vi "test_PhotonPoseEstimator_lowestAmbiguity.vi"(8 "error in (no error)":errorcluster) -> (0 "error out":errorcluster, 3 "Test Passed":bool)   [LabVIEW 2019]
uses:
  <vilib>/Rock Robotics/WPI/ThirdParty/PhotonVisionLib/TypeDef/PhotonEstimatedRobotPoseType.ctl
  <vilib>/Rock Robotics/WPI/ThirdParty/JAS_Junk/TrajLib/TypeDef/POSE3D.ctl
  <vilib>/Rock Robotics/WPI/ThirdParty/JAS_Junk/TrajLib/TypeDef/TRANSLATION3D.ctl
  <vilib>/Rock Robotics/WPI/ThirdParty/JAS_Junk/TrajLib/TypeDef/ROTATION3D.ctl
  <vilib>/Rock Robotics/WPI/ThirdParty/JAS_Junk/TrajLib/TypeDef/QUATERNION.ctl
  <vilib>/Rock Robotics/WPI/ThirdParty/PhotonVisionLib/TypeDef/PhotonPoseStrategy_ENUM.ctl
  <vilib>/Rock Robotics/WPI/ThirdParty/JAS_Junk/TrajLib/VI/Translation3d_Create_Default.vi
  <vilib>/Rock Robotics/WPI/ThirdParty/JAS_Junk/TrajLib/VI/Rotation3d_Create_Default.vi
  <vilib>/Rock Robotics/WPI/ThirdParty/JAS_Junk/TrajLib/VI/Quaternion_New.vi
  <vilib>/Rock Robotics/WPI/ThirdParty/PhotonVisionLib/SubVI/PhotonPipelineResult_HasTargets.vi
  <vilib>/Rock Robotics/WPI/ThirdParty/PhotonVisionLib/SubVI/PhotonEstimatedRobotPose_New.vi
  <vilib>/Rock Robotics/WPI/ThirdParty/PhotonVisionLib/SubVI/PhotonPipelineResult_GetTargets.vi
  <vilib>/Rock Robotics/WPI/ThirdParty/PhotonVisionLib/SubVI/PhotonTrackedTarget_GetPoseAmbiguity.vi
  <vilib>/Rock Robotics/WPI/ThirdParty/PhotonVisionLib/SubVI/PhotonTrackedTarget_GetFiducialId.vi
  <vilib>/Rock Robotics/WPI/ThirdParty/PhotonVisionLib/SubVI/PhotonPoseEstimator_GetFieldTags.vi
  <vilib>/Rock Robotics/WPI/ThirdParty/JAS_Junk/TrajLib/VI/AprilTagFieldLayout_GetTagPose.vi
  <vilib>/Rock Robotics/WPI/ThirdParty/JAS_Junk/TrajLib/VI/Pose3d_TransformBy.vi
  <vilib>/Rock Robotics/WPI/ThirdParty/PhotonVisionLib/SubVI/PhotonTrackedTarget_GetBestCameraToTarget.vi
  <vilib>/Rock Robotics/WPI/ThirdParty/JAS_Junk/TrajLib/VI/Transform3d_Inverse.vi
  <vilib>/Rock Robotics/WPI/ThirdParty/PhotonVisionLib/SubVI/PhotonPoseEstimator_GetHighestAmbiguity.vi
  <vilib>/Rock Robotics/WPI/ThirdParty/PhotonVisionLib/SubVI/PhotonPipelineResult_GetTimeStampSecs.vi
  <vilib>/Rock Robotics/WPI/ThirdParty/PhotonVisionLib/SubVI/PhotonPoseEstimator_GetRobotToCamera.vi
  <vilib>/Rock Robotics/WPI/ThirdParty/PhotonVisionLib/SubVI/PhotonPoseEstimator_GetEmptyPose.vi
  <vilib>/Rock Robotics/WPI/ThirdParty/JAS_Junk/TrajLib/VI/Quaternion_New_Default.vi
  <vilib>/Rock Robotics/WPI/ThirdParty/JAS_Junk/TrajLib/VI/AprilTag_GetAll.vi
  <vilib>/Rock Robotics/WPI/ThirdParty/JAS_Junk/TrajLib/VI/Pose3d_RelativeTo.vi
  <vilib>/Rock Robotics/WPI/ThirdParty/JAS_Junk/TrajLib/VI/Pose3d_getTranslation3d.vi
  <vilib>/Rock Robotics/WPI/ThirdParty/JAS_Junk/TrajLib/VI/Pose3d_getRotation3d.vi
  <vilib>/Rock Robotics/WPI/ThirdParty/JAS_Junk/TrajLib/VI/Transform3d_GetTranslation3d.vi
  <vilib>/Rock Robotics/WPI/ThirdParty/JAS_Junk/TrajLib/VI/Transform3d_GetRotation3d.vi
  <vilib>/Rock Robotics/WPI/ThirdParty/JAS_Junk/TrajLib/VI/Translation3d_Plus.vi
  <vilib>/Rock Robotics/WPI/ThirdParty/JAS_Junk/TrajLib/VI/Translation3d_RotateBy.vi
  <vilib>/Rock Robotics/WPI/ThirdParty/JAS_Junk/TrajLib/VI/Pose3d_New_Trans3dRot3d.vi
  <vilib>/Rock Robotics/WPI/ThirdParty/JAS_Junk/TrajLib/VI/Rotation3d_Plus.vi
  <vilib>/Rock Robotics/WPI/ThirdParty/JAS_Junk/TrajLib/VI/Translation3d_ToTranslation2d.vi
  <vilib>/Rock Robotics/WPI/ThirdParty/JAS_Junk/TrajLib/VI/Rotation3d_ToRotation2d.vi
  <vilib>/Rock Robotics/WPI/ThirdParty/JAS_Junk/TrajLib/Transform2d_Create_TransRot.vi
  <vilib>/Rock Robotics/WPI/ThirdParty/JAS_Junk/TrajLib/VI/Rotation3d_UnaryMinus.vi
  <vilib>/Rock Robotics/WPI/ThirdParty/JAS_Junk/TrajLib/VI/Translation3d_UnaryMinus.vi
  <vilib>/Rock Robotics/WPI/ThirdParty/JAS_Junk/TrajLib/VI/Rotation3d_Create_AxisAngle.vi
  <vilib>/Rock Robotics/WPI/ThirdParty/JAS_Junk/TrajLib/VI/Pose3d_New.vi
  <vilib>/Rock Robotics/WPI/ThirdParty/JAS_Junk/TrajLib/VI/Transform3d_Create_Pose3dPose3d.vi
  <vilib>/Rock Robotics/WPI/ThirdParty/JAS_Junk/TrajLib/VI/Rotation3d_GetQuaterion.vi
  <vilib>/Rock Robotics/WPI/ThirdParty/JAS_Junk/TrajLib/VI/Quaternion_Times.vi
  <vilib>/Rock Robotics/WPI/ThirdParty/JAS_Junk/TrajLib/VI/Quaternion_Inverse.vi
  <vilib>/Rock Robotics/WPI/ThirdParty/JAS_Junk/TrajLib/VI/Quaternion_Get_All.vi
  <vilib>/Rock Robotics/WPI/ThirdParty/JAS_Junk/TrajLib/VI/Rotation3d_RotateBy.vi
  <vilib>/Rock Robotics/WPI/ThirdParty/JAS_Junk/TrajLib/Translation2d_Create.vi
  <vilib>/Rock Robotics/WPI/ThirdParty/JAS_Junk/TrajLib/Rotation2d_CreateAngle.vi
  <vilib>/Rock Robotics/WPI/ThirdParty/JAS_Junk/TrajLib/VI/Rotation3d_GetXYZ.vi
  <vilib>/Rock Robotics/WPI/ThirdParty/JAS_Junk/TrajLib/VI/Rotation3d_Create_Quaternion.vi
  <vilib>/Rock Robotics/WPI/ThirdParty/JAS_Junk/TrajLib/VI/Vector_Norm.vi
  <vilib>/Rock Robotics/WPI/ThirdParty/JAS_Junk/TrajLib/VecBuilder_ArrayBy1Fill.vi
  <vilib>/Rock Robotics/WPI/ThirdParty/JAS_Junk/TrajLib/VI/Translation3d_Minus.vi
  <vilib>/Rock Robotics/WPI/ThirdParty/JAS_Junk/TrajLib/VI/Rotation3d_Minus.vi
  <vilib>/Rock Robotics/WPI/ThirdParty/JAS_Junk/TrajLib/VI/Quaternion_Normalize.vi
  <vilib>/Rock Robotics/WPI/ThirdParty/JAS_Junk/TrajLib/MatBuilder_Create.vi
  <vilib>/Rock Robotics/WPI/ThirdParty/JAS_Junk/TrajLib/Trajectory_Library.lvlib
  <vilib>/Rock Robotics/WPI/ThirdParty/PhotonVisionLib/PhotonVisionLib.lvlib
panel:
  out "Pos Found":bool
  out "PhotonEstimatedRobotPose":T1={"EstimatedPose"={"Translation3d"={"X"=0.0, "Y"=0.0, "Z"=0.0}, "Rotation3d"={"Q_quaternion"={"R"=1.0, "V"=[0.0, 0.0, 0.0]}}}, "TimeStamp_Seconds"=0.0} {"EstimatedPose"."Translation3d"."Z" format="%14.3f"; "EstimatedPose"."Translation3d"."Y" format="%14.3f"; "EstimatedPose"."Translation3d"."X" format="%14.3f"}
  out "Test 0 Passed":bool
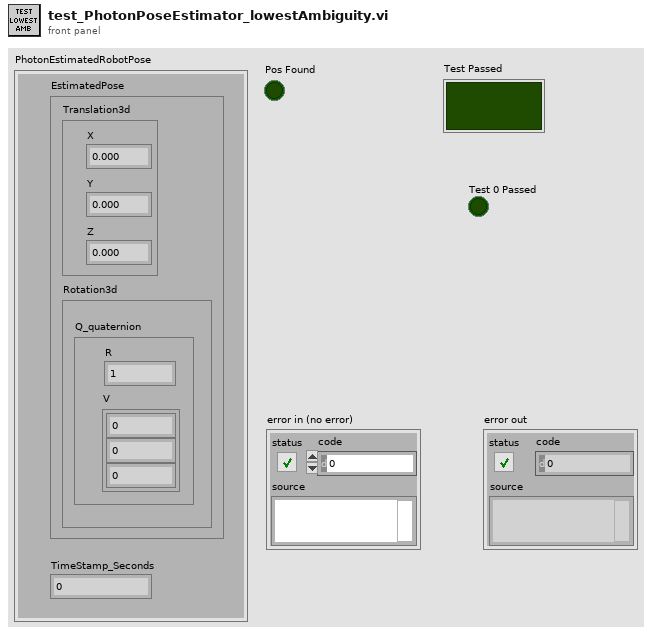
[diagram p1: front panel]
types:
  T1 = typedef "PhotonVisionLib.lvlib/PhotonEstimatedRobotPoseType.ctl" = cluster{"EstimatedPose":T2, "TimeStamp_Seconds":dbl}
  T2 = typedef "Trajectory_Library.lvlib/POSE3D.ctl" = cluster{"Translation3d":T3, "Rotation3d":T4}
  T3 = typedef "Trajectory_Library.lvlib/TRANSLATION3D.ctl" = cluster{"X":dbl, "Y":dbl, "Z":dbl}
  T4 = typedef "Trajectory_Library.lvlib/ROTATION3D.ctl" = cluster{"Q_quaternion":T5}
  T5 = typedef "Trajectory_Library.lvlib/QUATERNION.ctl" = cluster{"R":dbl, "V":dbl[]}
  T6 = typedef "PhotonVisionLib.lvlib/PhotonPoseStrategy_ENUM.ctl" = enum16{"LOWEST_AMBIGUITY", "CLOSEST_TO_CAMERA_HEIGHT", "CLOSEST_TO_REFERENCE_POSE", "CLOSEST_TO_LAST_POSE", "AVERAGE_BEST_TARGETS"}
  T7 = typedef "PhotonVisionLib.lvlib/TargetCornerType.ctl" = cluster{"X":dbl, "Y":dbl}
  T8 = typedef "Trajectory_Library.lvlib/AprilTagFieldLayout.ctl" = cluster{"AprilTagMap":map{i32, T9}, "FieldLength":dbl, "FieldWidth":dbl, "OriginPosition ":T10, "OriginPose3d":T2}
  T9 = typedef "Trajectory_Library.lvlib/AprilTag.ctl" = cluster{"ID":i32, "POSE3D":T2}
  T10 = typedef "Trajectory_Library.lvlib/AprilTagFieldLayoutOrignPosition_ENUM.ctl" = enum16{"kBlueAllianceWallRightSide,", "kRedAllianceWallRightSide,"}
  T11 = typedef "Trajectory_Library.lvlib/TRANSFORM3D.ctl" = cluster{"TRANSLATION3D":T3, "ROTATION3D":T4, "XF":bool}
  T12 = typedef "PhotonVisionLib.lvlib/PhotonTrackedTargetType.ctl" = cluster{"Yaw":dbl, "Pitch":dbl, "Area":dbl, "Skew":dbl, "MinAreaRectCorners":T7[], "BestCameraToTarget":T11, "FiiducialId":i32, "AltCameraToTarget":T11, "PoseAmbiguity":dbl, "DetectedCorners":T7[]}
  T13 = typedef "PhotonVisionLib.lvlib/PhotonPipelineResultType.ctl" = cluster{"TargetCount":i32, "Latency_MilliSec":dbl, "Targets":T12[], "TimeStampSec":dbl}
  T14 = typedef "PhotonVisionLib.lvlib/PhotonPoseEstimatorType.ctl" = cluster{"LastPose":T2, "ReferencePose":T2, "FieldTags":T8, "PhotonPoseStrategy":T6, "Camera":string, "RobotToCamera":T11, "ReportedErrors":dbl[], "HighestAmbiguity":dbl}
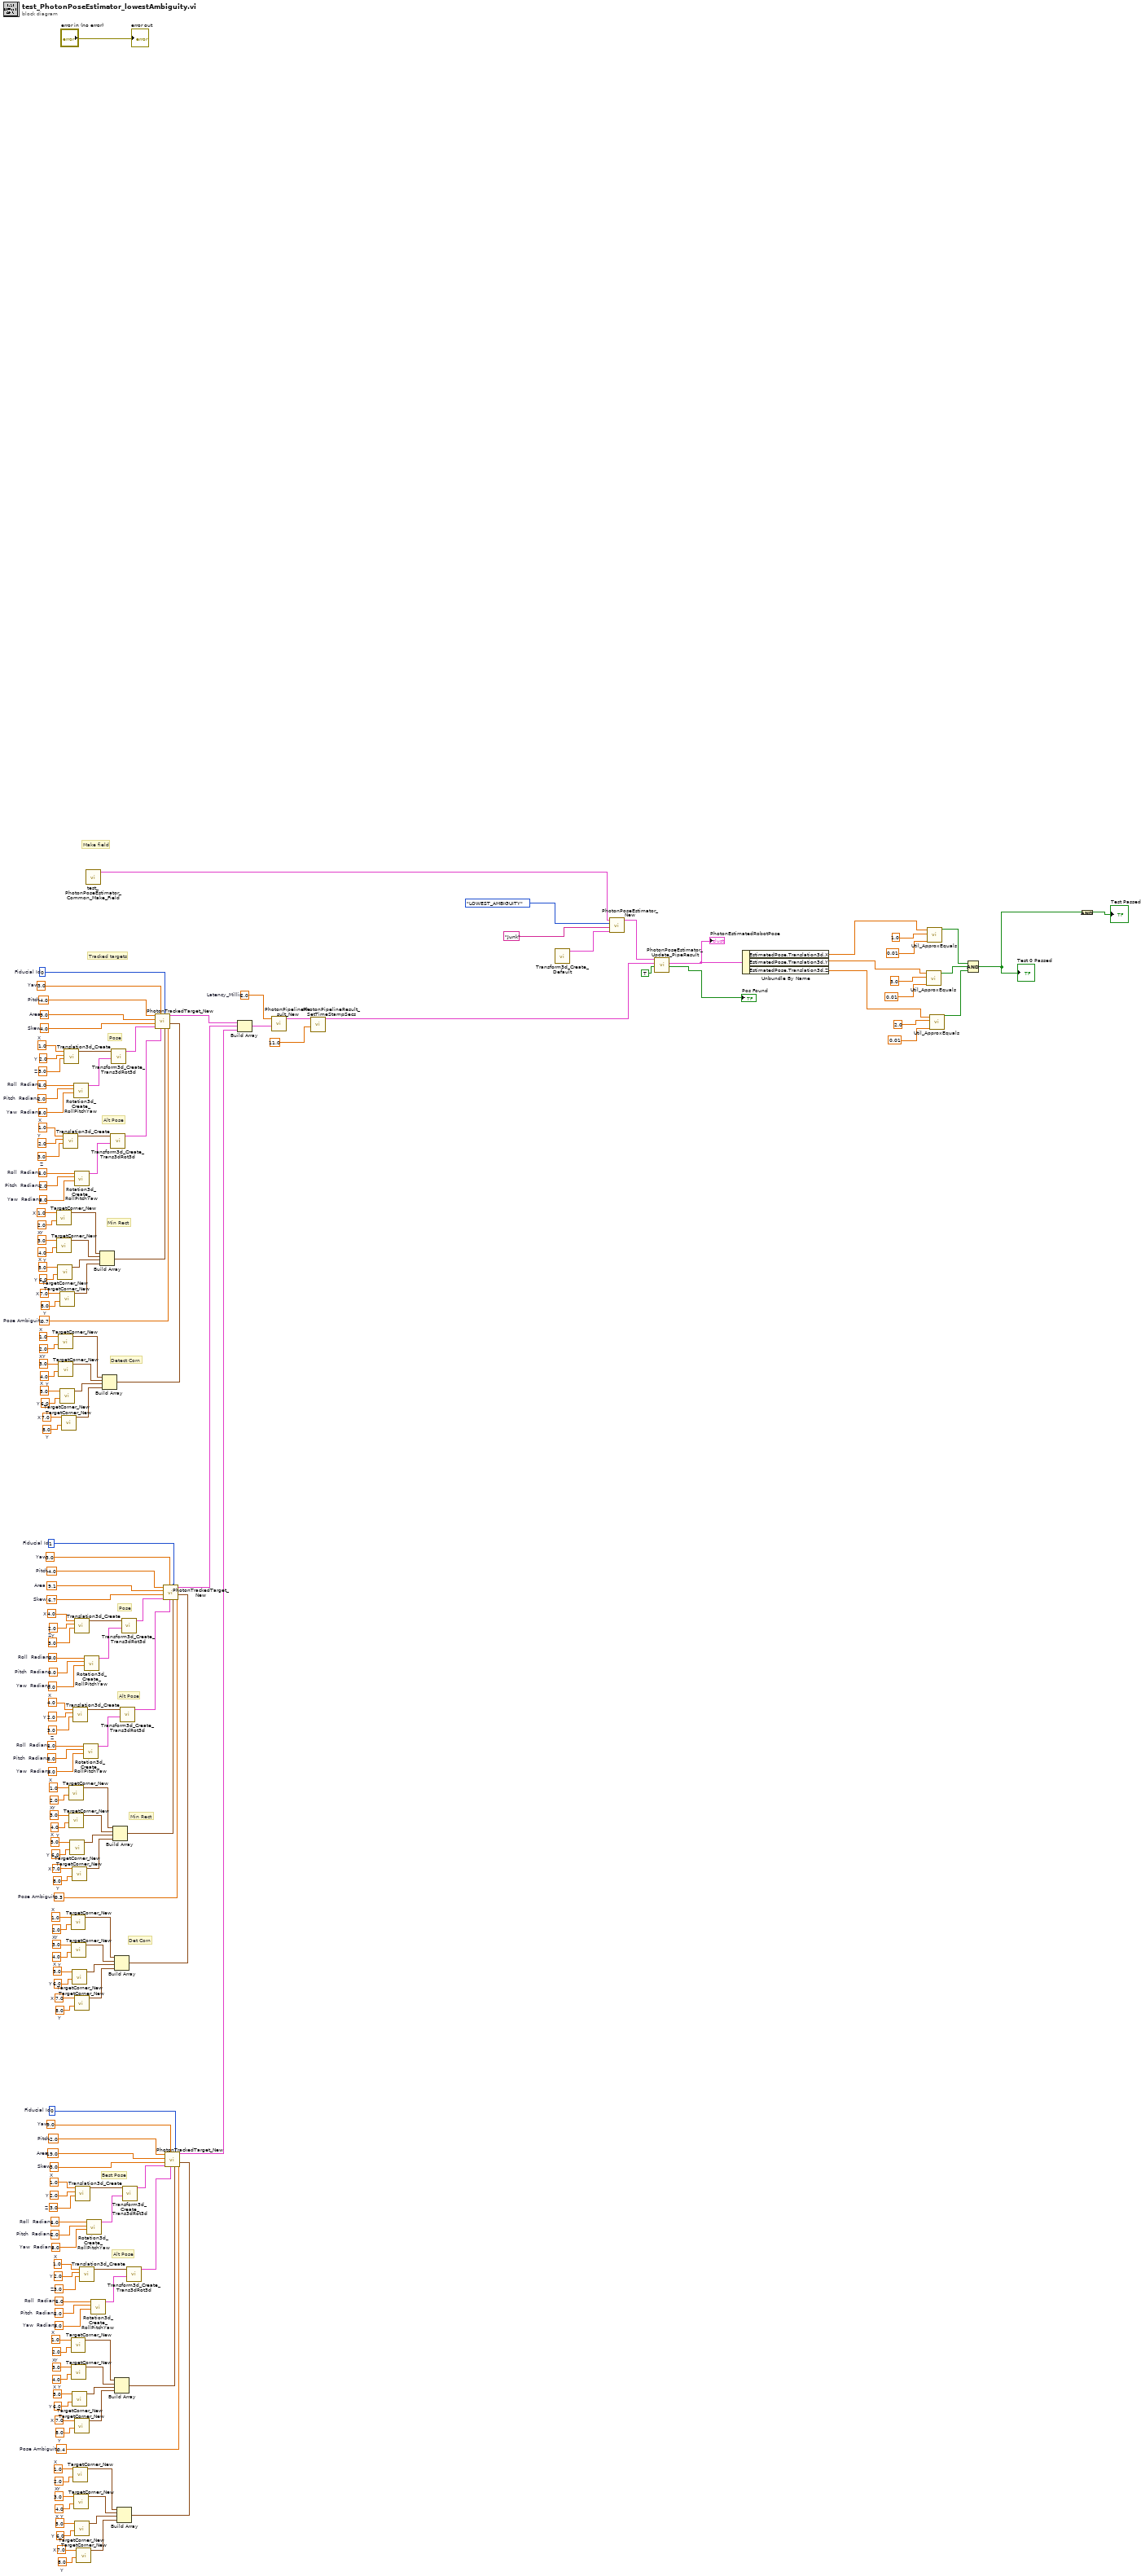
[diagram p0: block diagram]
diagram:
  w22 = 2.0  # Latency_Millis
  w32 = 1.0  # Roll  Radians
  w31 = 2.0  # Pitch  Radians
  w30 = 3.0  # Yaw  Radians
  w35 = 3.0  # Z
  w34 = 1.0  # X
  w33 = 2.0  # Y
  w40 = 1.0  # Roll  Radians
  w39 = 2.0  # Pitch  Radians
  w38 = 3.0  # Yaw  Radians
  w43 = 3.0  # Z
  w42 = 1.0  # X
  w41 = 2.0  # Y
  w50 = 7.0  # X
  w51 = 8.0  # Y
  w52 = 5.0  # X
  w53 = 6.0  # Y
  w54 = 3.0  # X
  w55 = 4.0  # Y
  w56 = 1.0  # X
  w57 = 2.0  # Y
  w62 = 7.0  # X
  w63 = 8.0  # Y
  w64 = 5.0  # X
  w65 = 6.0  # Y
  w66 = 3.0  # X
  w67 = 4.0  # Y
  w68 = 1.0  # X
  w69 = 2.0  # Y
  w70 = -2.0  # Pitch
  w71 = 19.0  # Area
  w72 = 3.0  # Skew
  w73 = 0  # Fiducial Id
  w74 = 0.4  # Pose Ambiguity
  w75 = 9.0  # Yaw
  w82 = 0.0  # Roll  Radians
  w81 = 0.0  # Pitch  Radians
  w80 = 0.0  # Yaw  Radians
  w85 = 3.0  # Z
  w84 = 4.0  # X
  w83 = 2.0  # Y
  w90 = 1.0  # Roll  Radians
  w89 = 5.0  # Pitch  Radians
  w88 = 3.0  # Yaw  Radians
  w93 = 3.0  # Z
  w92 = 4.0  # X
  w91 = 2.0  # Y
  w100 = 7.0  # X
  w101 = 8.0  # Y
  w102 = 5.0  # X
  w103 = 6.0  # Y
  w104 = 3.0  # X
  w105 = 4.0  # Y
  w106 = 1.0  # X
  w107 = 2.0  # Y
  w112 = 7.0  # X
  w113 = 8.0  # Y
  w114 = 5.0  # X
  w115 = 6.0  # Y
  w116 = 3.0  # X
  w117 = 4.0  # Y
  w118 = 1.0  # X
  w119 = 2.0  # Y
  w120 = -4.0  # Pitch
  w121 = 9.1  # Area
  w122 = 6.7  # Skew
  w123 = 1  # Fiducial Id
  w124 = 0.3  # Pose Ambiguity
  w125 = 3.0  # Yaw
  w132 = 1.0  # Roll  Radians
  w131 = 2.0  # Pitch  Radians
  w130 = 3.0  # Yaw  Radians
  w135 = 3.0  # Z
  w134 = 1.0  # X
  w133 = 2.0  # Y
  w140 = 1.0  # Roll  Radians
  w139 = 2.0  # Pitch  Radians
  w138 = 3.0  # Yaw  Radians
  w143 = 3.0  # Z
  w142 = 1.0  # X
  w141 = 2.0  # Y
  w150 = 7.0  # X
  w151 = 8.0  # Y
  w152 = 5.0  # X
  w153 = 6.0  # Y
  w154 = 3.0  # X
  w155 = 4.0  # Y
  w156 = 1.0  # X
  w157 = 2.0  # Y
  w162 = 7.0  # X
  w163 = 8.0  # Y
  w164 = 5.0  # X
  w165 = 6.0  # Y
  w166 = 3.0  # X
  w167 = 4.0  # Y
  w168 = 1.0  # X
  w169 = 2.0  # Y
  w170 = -4.0  # Pitch
  w171 = 9.0  # Area
  w172 = 4.0  # Skew
  w173 = 0  # Fiducial Id
  w174 = 0.7  # Pose Ambiguity
  w175 = 3.0  # Yaw
  # "Det Corn"
  # "Min Rect"
  # "Pose"
  # "Detect Corn"
  # "Min Rect"
  # "Tracked targets"
  # "Make field"
  # "Best Pose"
  # "Alt Pose"
  # "Alt Pose"
  # "Pose"
  # "Alt Pose"
  n1 = call <vilib>:"TargetCorner_New.vi"("Y"=w169, "X"=w168) -> ("TargetCorner"=w161:T7)  [unwired: 9 in]
  n2 = call <vilib>:"TargetCorner_New.vi"("Y"=w167, "X"=w166) -> ("TargetCorner"=w160:T7)  [unwired: 9 in]
  n3 = call <vilib>:"TargetCorner_New.vi"("Y"=w165, "X"=w164) -> ("TargetCorner"=w159:T7)  [unwired: 9 in]
  n4 = call <vilib>:"TargetCorner_New.vi"("Y"=w157, "X"=w156) -> ("TargetCorner"=w149:T7)  [unwired: 9 in]
  n5 = call <vilib>:"TargetCorner_New.vi"("Y"=w155, "X"=w154) -> ("TargetCorner"=w148:T7)  [unwired: 9 in]
  n6 = call <vilib>:"TargetCorner_New.vi"("Y"=w163, "X"=w162) -> ("TargetCorner"=w158:T7)  [unwired: 9 in]
  n7 = call <vilib>:"TargetCorner_New.vi"("Y"=w153, "X"=w152) -> ("TargetCorner"=w147:T7)  [unwired: 9 in]
  n8 = call <vilib>:"TargetCorner_New.vi"("Y"=w151, "X"=w150) -> ("TargetCorner"=w146:T7)  [unwired: 9 in]
  n9 = call <vilib>:"Translation3d_Create.vi"("Z"=w143, "Y"=w141, "X"=w142) -> ("TRANSLATION3D"=w137:T3)  [unwired: 8 in]
  n10 = call <vilib>:"Translation3d_Create.vi"("Z"=w135, "Y"=w133, "X"=w134) -> ("TRANSLATION3D"=w129:T3)  [unwired: 8 in]
  n11 = call <vilib>:"TargetCorner_New.vi"("Y"=w119, "X"=w118) -> ("TargetCorner"=w111:T7)  [unwired: 9 in]
  n12 = call <vilib>:"TargetCorner_New.vi"("Y"=w117, "X"=w116) -> ("TargetCorner"=w110:T7)  [unwired: 9 in]
  n13 = call <vilib>:"TargetCorner_New.vi"("Y"=w115, "X"=w114) -> ("TargetCorner"=w109:T7)  [unwired: 9 in]
  n14 = call <vilib>:"TargetCorner_New.vi"("Y"=w107, "X"=w106) -> ("TargetCorner"=w99:T7)  [unwired: 9 in]
  n15 = call <vilib>:"TargetCorner_New.vi"("Y"=w69, "X"=w68) -> ("TargetCorner"=w61:T7)  [unwired: 9 in]
  n16 = call <vilib>:"TargetCorner_New.vi"("Y"=w105, "X"=w104) -> ("TargetCorner"=w98:T7)  [unwired: 9 in]
  n17 = call <vilib>:"TargetCorner_New.vi"("Y"=w67, "X"=w66) -> ("TargetCorner"=w60:T7)  [unwired: 9 in]
  n18 = call <vilib>:"TargetCorner_New.vi"("Y"=w113, "X"=w112) -> ("TargetCorner"=w108:T7)  [unwired: 9 in]
  n19 = call <vilib>:"TargetCorner_New.vi"("Y"=w103, "X"=w102) -> ("TargetCorner"=w97:T7)  [unwired: 9 in]
  n20 = call <vilib>:"TargetCorner_New.vi"("Y"=w65, "X"=w64) -> ("TargetCorner"=w59:T7)  [unwired: 9 in]
  n21 = call <vilib>:"Translation3d_Create.vi"("Z"=w93, "Y"=w91, "X"=w92) -> ("TRANSLATION3D"=w87:T3)  [unwired: 8 in]
  n22 = call <vilib>:"TargetCorner_New.vi"("Y"=w57, "X"=w56) -> ("TargetCorner"=w49:T7)  [unwired: 9 in]
  n23 = call <vilib>:"Rotation3d_Create_RollPitchYaw.vi"("Yaw"=w130, "Pitch"=w131, "Roll"=w132) -> ("Rotation3d"=w128:T4)  [unwired: 8 in]
  n24 = call <vilib>:"TargetCorner_New.vi"("Y"=w55, "X"=w54) -> ("TargetCorner"=w48:T7)  [unwired: 9 in]
  n25 = call <vilib>:"Rotation3d_Create_RollPitchYaw.vi"("Yaw"=w138, "Pitch"=w139, "Roll"=w140) -> ("Rotation3d"=w136:T4)  [unwired: 8 in]
  n26 = call <vilib>:"Translation3d_Create.vi"("Z"=w85, "Y"=w83, "X"=w84) -> ("TRANSLATION3D"=w79:T3)  [unwired: 8 in]
  n27 = call <vilib>:"TargetCorner_New.vi"("Y"=w101, "X"=w100) -> ("TargetCorner"=w96:T7)  [unwired: 9 in]
  n28 = call <vilib>:"TargetCorner_New.vi"("Y"=w63, "X"=w62) -> ("TargetCorner"=w58:T7)  [unwired: 9 in]
  n29 = call <vilib>:"TargetCorner_New.vi"("Y"=w53, "X"=w52) -> ("TargetCorner"=w47:T7)  [unwired: 9 in]
  n30 = call <vilib>:"Translation3d_Create.vi"("Z"=w35, "Y"=w33, "X"=w34) -> ("TRANSLATION3D"=w29:T3)  [unwired: 8 in]
  n31 = call <vilib>:"TargetCorner_New.vi"("Y"=w51, "X"=w50) -> ("TargetCorner"=w46:T7)  [unwired: 9 in]
  n32 = call <vilib>:"Translation3d_Create.vi"("Z"=w43, "Y"=w41, "X"=w42) -> ("TRANSLATION3D"=w37:T3)  [unwired: 8 in]
  n33 = call <vilib>:"Rotation3d_Create_RollPitchYaw.vi"("Yaw"=w88, "Pitch"=w89, "Roll"=w90) -> ("Rotation3d"=w86:T4)  [unwired: 8 in]
  n34 = call <vilib>:"Rotation3d_Create_RollPitchYaw.vi"("Yaw"=w80, "Pitch"=w81, "Roll"=w82) -> ("Rotation3d"=w78:T4)  [unwired: 8 in]
  n35 = call "test_PhotonPoseEstimator_Common_Make_Field.vi"() -> ("AprilTagFieldLayout"=w18:T8)  [unwired: 11 in]
  n36 = call <vilib>:"Rotation3d_Create_RollPitchYaw.vi"("Yaw"=w30, "Pitch"=w31, "Roll"=w32) -> ("Rotation3d"=w28:T4)  [unwired: 8 in]
  n37 = call <vilib>:"Rotation3d_Create_RollPitchYaw.vi"("Yaw"=w38, "Pitch"=w39, "Roll"=w40) -> ("Rotation3d"=w36:T4)  [unwired: 8 in]
  n38 = Build Array(w161, w160, w159, w158) -> (w145:T7[])
  n39 = Build Array(w149, w148, w147, w146) -> (w144:T7[])
  n40 = call <vilib>:"Transform3d_Create_Trans3dRot3d.vi"("Rotation3d"=w136, "Translation3d"=w137) -> ("Transform3d"=w126:T11)  [unwired: 9 in]
  n41 = call <vilib>:"Transform3d_Create_Trans3dRot3d.vi"("Rotation3d"=w128, "Translation3d"=w129) -> ("Transform3d"=w127:T11)  [unwired: 9 in]
  n42 = Build Array(w111, w110, w109, w108) -> (w95:T7[])
  n43 = Build Array(w99, w98, w97, w96) -> (w94:T7[])
  n44 = Build Array(w61, w60, w59, w58) -> (w45:T7[])
  n45 = Build Array(w49, w48, w47, w46) -> (w44:T7[])
  n46 = call <vilib>:"Transform3d_Create_Trans3dRot3d.vi"("Rotation3d"=w86, "Translation3d"=w87) -> ("Transform3d"=w76:T11)  [unwired: 9 in]
  n47 = call <vilib>:"Transform3d_Create_Trans3dRot3d.vi"("Rotation3d"=w78, "Translation3d"=w79) -> ("Transform3d"=w77:T11)  [unwired: 9 in]
  n48 = call <vilib>:"Transform3d_Create_Trans3dRot3d.vi"("Rotation3d"=w28, "Translation3d"=w29) -> ("Transform3d"=w27:T11)  [unwired: 9 in]
  n49 = call <vilib>:"Transform3d_Create_Trans3dRot3d.vi"("Rotation3d"=w36, "Translation3d"=w37) -> ("Transform3d"=w26:T11)  [unwired: 9 in]
  n50 = call <vilib>:"PhotonTrackedTarget_New.vi"("Pose Ambiguity"=w174, "DetectedCorners"=w144, "MinAreaRectCorners"=w145, "Fiducial Id"=w173, "AltCameraToTarget"=w126, "Yaw"=w175, "BestCameraToTarget"=w127, "Skew"=w172, "Area"=w171, "Pitch"=w170) -> ("TrackedTarget"=w25:T12)  [unwired: 1 in]
  n51 = call <vilib>:"PhotonTrackedTarget_New.vi"("Pose Ambiguity"=w124, "DetectedCorners"=w94, "MinAreaRectCorners"=w95, "Fiducial Id"=w123, "AltCameraToTarget"=w76, "Yaw"=w125, "BestCameraToTarget"=w77, "Skew"=w122, "Area"=w121, "Pitch"=w120) -> ("TrackedTarget"=w24:T12)  [unwired: 1 in]
  n52 = call <vilib>:"PhotonTrackedTarget_New.vi"("Pose Ambiguity"=w74, "DetectedCorners"=w44, "MinAreaRectCorners"=w45, "Fiducial Id"=w73, "AltCameraToTarget"=w26, "Yaw"=w75, "BestCameraToTarget"=w27, "Skew"=w72, "Area"=w71, "Pitch"=w70) -> ("TrackedTarget"=w23:T12)  [unwired: 1 in]
  n53 = Build Array(w25, w24, w23) -> (w21:T12[])
  n54 = call <vilib>:"PhotonPipelineResult_New.vi"("TrackedTargets"=w21, "Latency_Millis"=w22) -> ("PhotonPipelineResult"=w20:T13)  [unwired: 9 in]
  n55 = call <vilib>:"PhotonPipelineResult_SetTimeStampSecs.vi"("TimeStampSec"=11.0, "PhotonPipelineResult"=w20) -> ("Out PhotonPipelineResult"=w4:T13)  [unwired: 9 in]
  n56 = call <vilib>:"Transform3d_Create_Default.vi"() -> ("Transform3d"=w15:T11)  [unwired: 11 in]
  n57 = call <vilib>:"PhotonPoseEstimator_New.vi"("RobotToCamera"=w15, "Camera"="Junk", "Strategy"=PhotonPoseStrategy_ENUM."LOWEST_AMBIGUITY", "AprilTagFieldLayout"=w18) -> ("PhotonPoseEstimator"=w5:T14)  [unwired: 7 in]
  n58 = call <vilib>:"PhotonPoseEstimator_Update_PipeResult.vi"("Has Results"=TRUE, "PipelineResult"=w4, "PhotonPoseEstimator"=w5) -> ("Pos Found"=→"Pos Found":bool, "PhotonEstimatedRobotPose"=w2:T1)  [unwired: 6 in, 1 out]
  "PhotonEstimatedRobotPose" <- w2
  n59 = Unbundle By Name(w2) -> ("EstimatedPose.Translation3d.X"=w8:dbl, "EstimatedPose.Translation3d.Y"=w7:dbl, "EstimatedPose.Translation3d.Z"=w6:dbl)
  n60 = call <vilib>:"Util_ApproxEquals.vi"("Tolerance"=0.01, "Value 2"=3.0, "Value 1"=w7) -> ("ApproxEquals"=w10:bool)  [unwired: 8 in]
  n61 = call <vilib>:"Util_ApproxEquals.vi"("Tolerance"=0.01, "Value 2"=1.0, "Value 1"=w8) -> ("ApproxEquals"=w178:bool)  [unwired: 8 in]
  n62 = call <vilib>:"Util_ApproxEquals.vi"("Tolerance"=0.01, "Value 2"=2.0, "Value 1"=w6) -> ("ApproxEquals"=w9:bool)  [unwired: 8 in]
  n63 = Compound Arithmetic op=AND(w178, w10, w9) -> (w176:bool)
  "Test 0 Passed" <- w176
  n64 = Compound Arithmetic op=AND(w176) -> (→"Test Passed":bool)
  "error out" <- "error in (no error)"
